vi "Get Used Memory.vi"(8 "error in (no error)":errorcluster, 11 "KD Tree in":refnum<class "KD Tree.lvclass">) -> (0 "error out":errorcluster, 2 "Bytes":i32, 3 "KD Tree out":refnum<class "KD Tree.lvclass">)   [LabVIEW 2020, in "KD Tree.lvlib" / "KD Tree.lvclass"]
uses:
  KD Tree.lvclass
  KD Tree.lvlib
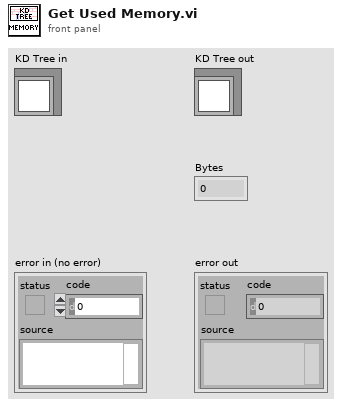
[diagram p1: front panel]
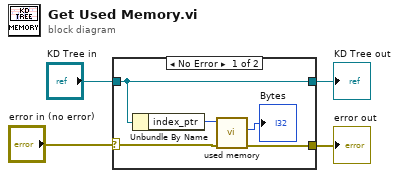
[diagram p0: block diagram]
diagram:
  n1 = case shown="No Error" "error in (no error)" {
    selector: "error in (no error)" -> [w7 w11]
    tunnel: [w6 w11] -> w3
    tunnel: [w9 w10] -> w1
    tunnel: "KD Tree in" -> [w9 w10]
    frame No Error {
      n2 = Unbundle By Name(w9) -> ("index_ptr"=w8:u64)
      n3 = call "used memory.vi"("error in (no error)"=w7, "index_ptr"=w8) -> ("error out"=w6:errorcluster, "Memory"=→"Bytes":i32)  [unwired: 7 in, 1 out]
    }
    frame Error {
    }
  }
  "error out" <- w3
  "KD Tree out" <- w1
